vi "Write VISA resource.vi"(8 "error in (no error)":errorcluster, 10 "VISA resource":refnum<visa-resource-name>, 11 "Yokogawa AQ6370D in":refnum<class "Yokogawa AQ6370D.lvclass">) -> (0 "error out":errorcluster, 3 "Yokogawa AQ6370D out":refnum<class "Yokogawa AQ6370D.lvclass">)   [LabVIEW 2018, in "Yokogawa AQ6370D.lvlib" / "Yokogawa AQ6370D.lvclass"]
uses:
  Yokogawa AQ6370D.lvclass
  Yokogawa AQ6370D.lvclass/Yokogawa AQ6370D.ctl
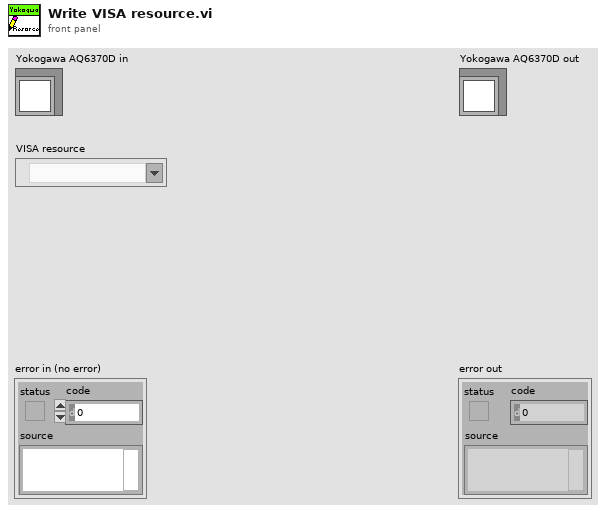
[diagram p1: front panel]
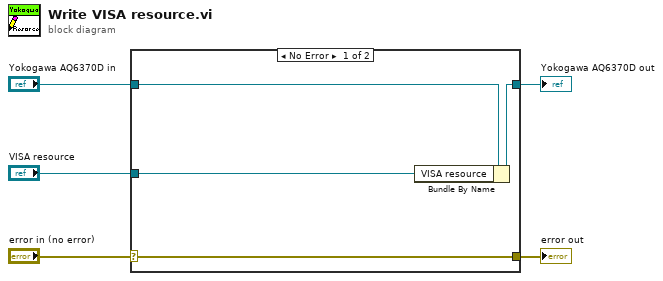
[diagram p0: block diagram]
diagram:
  n1 = case shown="No Error" "error in (no error)" {
    selector: "error in (no error)" -> [w9 w10]
    tunnel: [w9 w10] -> w4
    tunnel: [w7 w11] -> w2
    tunnel: "Yokogawa AQ6370D in" -> [w8 w11]
    tunnel: "VISA resource" -> [w6 _]
    frame No Error {
      n2 = Bundle By Name(cluster=w8, "VISA resource"=w6) -> (w7:refnum<class "Yokogawa AQ6370D.lvclass">)
    }
    frame Error {
    }
  }
  "error out" <- w4
  "Yokogawa AQ6370D out" <- w2
